vi "sc5511a_soft_front_panel.vi"() -> ()   [LabVIEW 2010]
panel:
  out "message":string="List/Sweep Mode Disabled"
  out "On":bool
  in  "stop":bool
  in  "Tab Control":T1(tab)
  in  "Spur Suppression":u8(ring) items=["Enabled", "Disabled"]
  in  "AutoLevel":u8(ring) items=["Enable", "Disable"]
  in  "Loop Gain":u8(ring) items=["Normal", "Low"]
  in  "Ref. Out Freq":u8(ring) items=["10 MHz", "100 MHz"]
  in  "Ref. Clock Source":u8(ring) items=["Internal 10 MHz", "Lock to External"]
  in  "RF1 Standby":bool
  in  "Lock Mode":u8(ring) items=["Harmonic Lock", "Frac-N Lock"]
  in  "ALC MODE":u8(ring) items=["Closed", "Opened"]
  in  "Power":sgl=30.0 min=-40 max=30 format="%.2f"
  in  "Interval (s)":u16=5
  in  "GetStatus":bool
  in  "Trigger":bool
  out "Device Status":T2={"Synth Mode"=1, "RF Out"=0, "Auto Level"=0, "ALC Mode"=1, "Standby"=1, "Rf RF Mode"=0, "List Mode State"=0, "RF2 Standby"=0, "Ref Lock Enable"=1, "Ext Ref Detected"=1, "Ref out mode"=1, "Main PLL"=1, "Crs PLL"=1, "Fine PLL"=1, "device accessed"=0, "Over Temp"=0, "MainLED"=FALSE, "CrsLED"=FALSE, "FineLED"=FALSE} {"Over Temp" items=["Normal", "Over Temp"]; "Ref out mode" items=["10 MHz", "100 MHz"]; "device accessed" items=["NO", "YES"]; "RF2 Standby" items=["Disabled", "Enabled"]; "Standby" items=["Disable", "Enabled"]; "Auto Level" items=["Enable", "Disable"]; "Ext Ref Detected" items=["Not Detected", "Detected"]; "Ref Lock Enable" items=["Disabled", "Enabled"]; "RF Out" items=["Disabled", "Enabled"]; "ALC Mode" items=["Closed", "Opened"]; "Rf RF Mode" items=["Single Tone", "List/Sweep"]; "Synth Mode" items=["Harmonic", "FracN"]; "List Mode State" items=["Not Triggered", "Triggered"]; "Main PLL" items=["NOT Locked", "Locked"]; "Crs PLL" items=["NOT Locked", "Locked"]; "Fine PLL" items=["NOT Locked", "Locked"]}
  in  "RF Frequency":dbl=2005000000.0 min=80000000.0 max=21000000000.0 step=1.0 format="%.9p"
  in  "RF Mode":u8(ring) items=["Single Tone", "List/Sweep"]
  in  "RF Enable":bool
  in  "RF2 Freq":sgl=6000.0 min=25 max=6000 step=25
  in  "RF2 Standby":bool
  in  "Set As Default":bool
  in  "Dwell Period (ms)":dbl=10.0 min=0.0 step=0.5 format="%.1f"
  in  "Sweep/List Cycles":u32
  in  "Sweep Freq Parameter":T3={"Start Frequency"=10040000000, "Stop Frequency"=10050000000, "Step Frequency"=100000} {"Step Frequency" max=6500000000 format="%.9p"; "Stop Frequency" max=21000000000 format="%.9p"; "Start Frequency" format="%.9p"}
  in  "List Mode Config":T4={"Sweep / List"=1, "Direction"=0, "Shape"=1, "Trigger Source"=1, "HW Trigger Mode"=0, "Return to Start"=0, "Trigger Out State"=1, "Trigger Out Behavior"=0} {"Trigger Out Behavior" items=["Trigger On Step", "Trigger On Cycle"]; "Trigger Out State" items=["Trigger Out Disable", "Trigger Out Enable"]; "Return to Start" items=["Stop at End", "Return to Start"]; "HW Trigger Mode" items=["Start/Stop", "Step"]; "Trigger Source" items=["Software", "Hardware"]; "Shape" items=["Sawtooth", "Triangle"]; "Direction" items=["Low to High", "High to Low"]; "Sweep / List" items=["List", "Sweep (start/stop/step)"]}
  in  "Load Config":bool
  in  "Save Buffer to EEPROM":bool
  in  "Read EEPROM to Buffer":bool
  in  "Download to Buffer":bool
  in  "Read From File":bool
  in  "Frequency List (2048 max)":u64[](array[numeric]) format="%.9p"
  out "message 2":string
  out "List Points":u32
  in  "SelfCal":bool
  out "Temperature":sgl=40.0 min=-30 max=120 format="%.1f"
  out "Device Info":T5={"Product SN"=268435879, "Hardware Rev"=2.0, "Firmware Rev"=2.0, "Manuf Date"={"Year"=14, "Month"=9, "Day"=10, "Hour"=10}} {"Firmware Rev" format="%.2g"; "Hardware Rev" format="%.2g"; "Product SN" format="%.0x"}
  out "error out":errorcluster
  # "MHz"
  # "Program will stop and the device will \nreinitialize after self calibration"
  # "DegC"
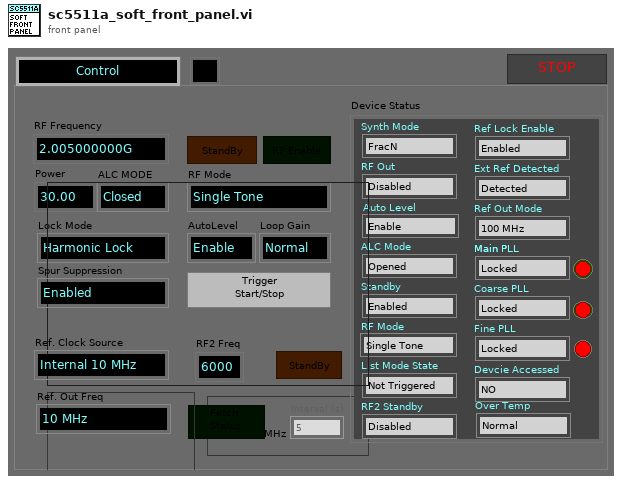
[diagram p1: front panel]
types:
  T1 = enum32{"Control", "Config Sweep/List", "List Entry", "Device Info"}
  T2 = cluster{"Synth Mode":u16, "RF Out":u16, "Auto Level":u16, "ALC Mode":u16, "Standby":u16, "Rf RF Mode":u16, "List Mode State":u16, "RF2 Standby":u16, "Ref Lock Enable":u16, "Ext Ref Detected":u16, "Ref out mode":u16, "Main PLL":u8, "Crs PLL":u8, "Fine PLL":u8, "device accessed":u16, "Over Temp":u16, "MainLED":bool, "CrsLED":bool, "FineLED":bool}
  T3 = cluster{"Start Frequency":u64, "Stop Frequency":u64, "Step Frequency":u64}
  T4 = cluster{"Sweep / List":u8, "Direction":u8, "Shape":u8, "Trigger Source":u8, "HW Trigger Mode":u8, "Return to Start":u8, "Trigger Out State":u8, "Trigger Out Behavior":u8}
  T5 = cluster{"Product SN":u32, "Hardware Rev":sgl, "Firmware Rev":sgl, "Manuf Date":cluster{"Year":u8, "Month":u8, "Day":u8, "Hour":u8}}
  T6 = cluster{"Product SN":u32, "Hardware Rev":sgl, "Firmware Rev":sgl, "Manuf Date":cluster{"Year":u32, "Month":u32, "Day":u32, "hour":u32}}
  T7 = enum32{"Control", "Config Sweep/List", "List Entry"}
  T8 = enum8{"Enabled", "Disabled", "Disabled and Grayed Out"}
  T9 = cluster{"Synth Mode":u16, "RF Out":u16, "Auto Power":u16, "ALC Mode":u16, "Standby":u16, "Rf RF Mode":u16, "List Mode State":u16, "RF2 Standby":u16, "Ref Lock Enable":u16, "Ext Ref Detected":u16, "Ref out mode":u16, "Main PLL":u8, "Crs PLL":u8, "Fine PLL":u8, "device accessed":u16, "Over Temp":u16, "MainLED":bool, "CrsLED":bool, "FineLED":bool}
  T10 = cluster{"Product SN":u32, "Hardware Rev":sgl, "Firmware Rev":sgl, "Manufacture Date":cluster{"Year":u8, "Month":u8, "Day":u8, "hour":u8}}
  T11 = cluster{"List Mode Config":cluster{"List/SSS":u8, "Direction":u8, "Shape":u8, "Trigger Source":u8, "HW Trigger Mode":u8, "Return to Start":u8, "Trigger Out State":u8, "Trigger Out Behavior":u8}, "Operate Status":cluster{"Lock Mode":u8, "Loop Gain":u8, "Device Accessed":u8, "RF2 Standby":u8, "RF1 Standby":u8, "AutoPwrLevel":u8, "AlcMode":u8, "RFOutState":u8, "Ref Lock Enable":u8, "ExtRefDetected":u8, "RefOutSelect":u8, "ListRuning":u8, "RF Mode":u8, "OverTempStatus":u8, "Harmonic SS":u8}, "PLL Status":cluster{"Sum PLL":u8, "Crs PLL":u8, "Fine PLL":u8, "Crs Ref PLL":u8, "Crs assist PLL":u8, "Ref Clk PLL":u8, "Clk 10 PLL":u8, "Lo2 PLL":u8}}
  T12 = cluster{"RF1 Freq":u64, "Sweep Start Freq":u64, "Sweep Stop Freq":u64, "Sweep Step Freq":u64, "Sweep dwell time (.5ms)":u32, "Sweep Cycles":u32, "List Buffer Points":u32, "RF1 Level (dBm)":sgl, "RF2 freq":u16}
  T13 = cluster{"List/SSS":u8, "Direction":u8, "Shape":u8, "Trigger Source":u8, "HW Trigger Mode":u8, "Return to Start":u8, "Trigger Out State":u8, "Trigger Out Behavior":u8}
  T14 = cluster{"Sweep Start Freq":u64, "Sweep Stop Freq":u64, "Sweep Step Freq":u64}
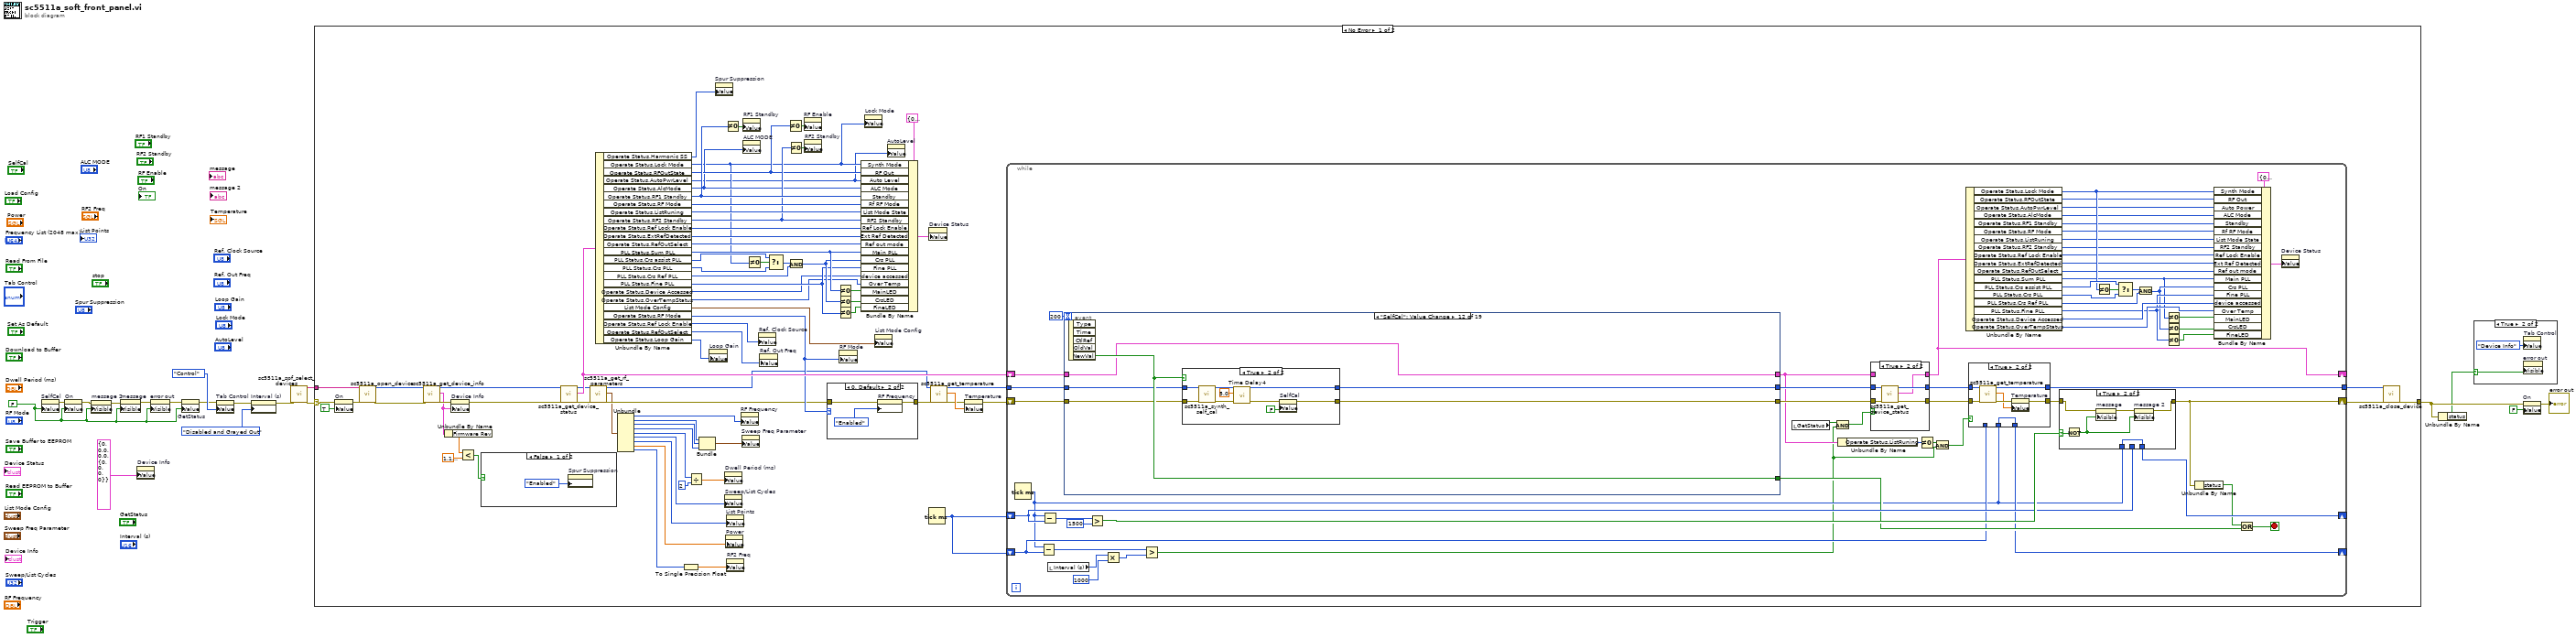
[diagram p0: block diagram]
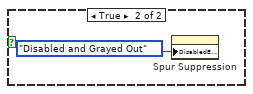
[diagram p3: hidden frame]
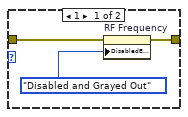
[diagram p4: hidden frame]
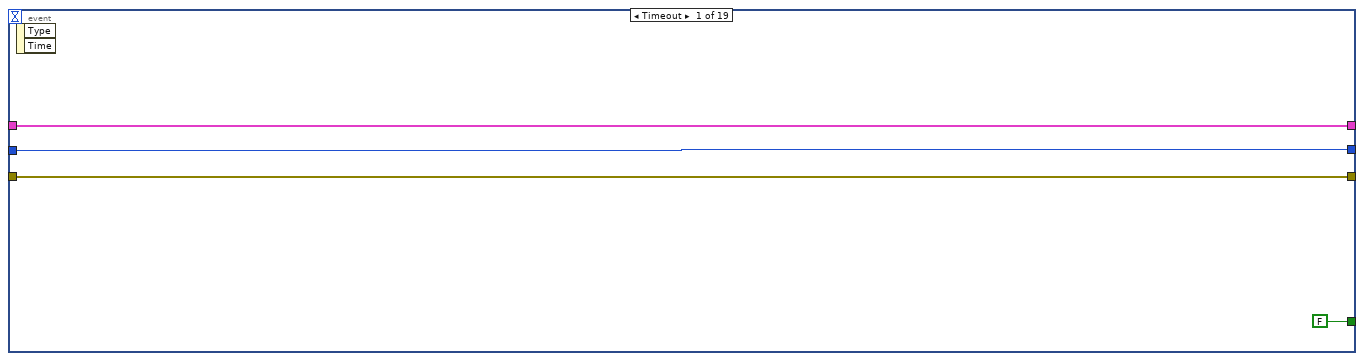
[diagram p8: hidden frame]
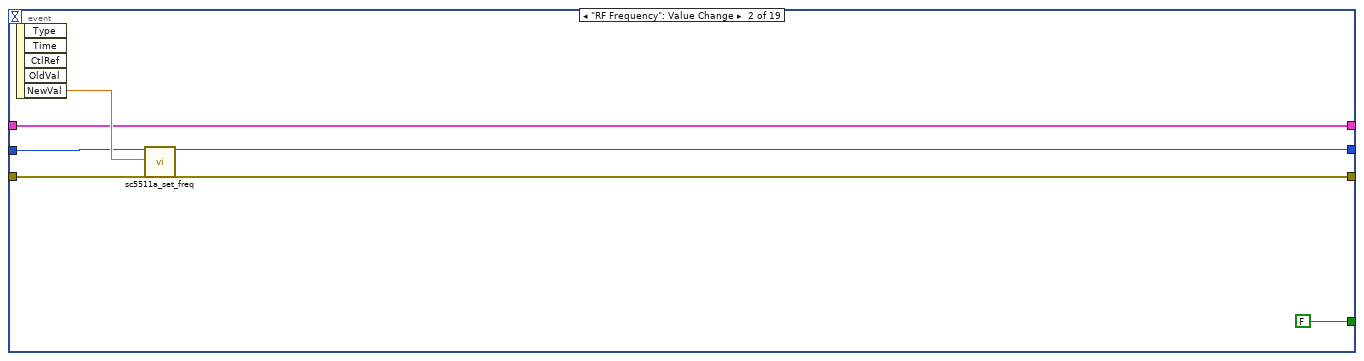
[diagram p9: hidden frame]
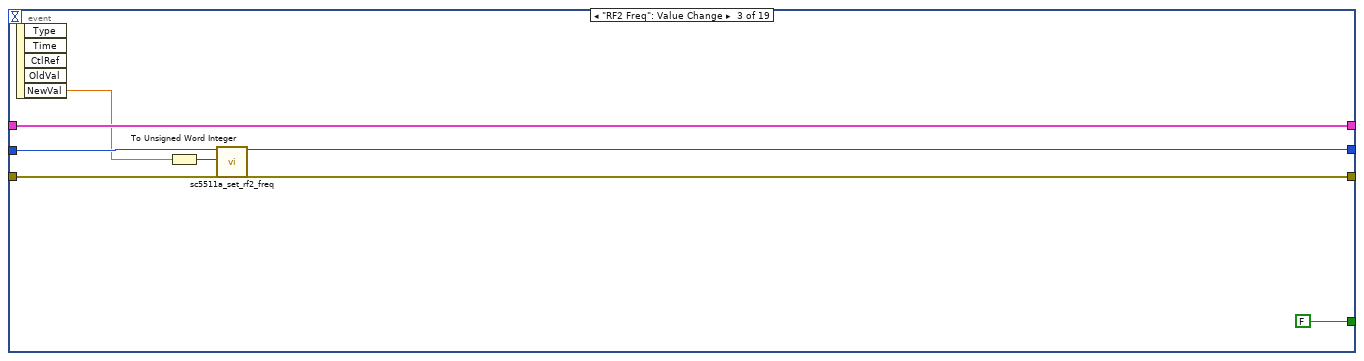
[diagram p10: hidden frame]
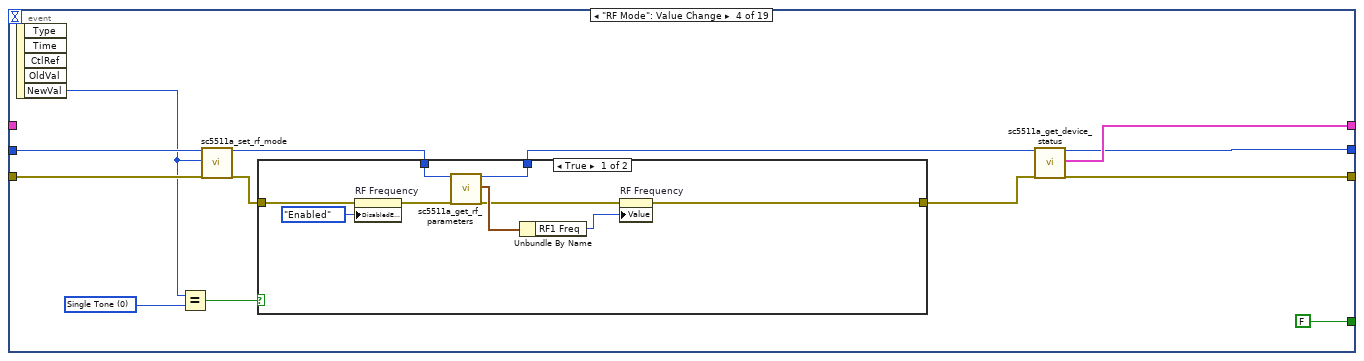
[diagram p11: hidden frame]
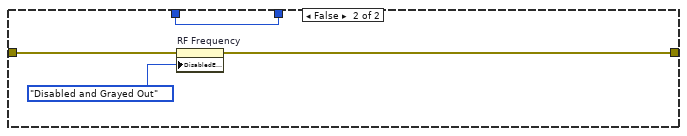
[diagram p12: hidden frame]
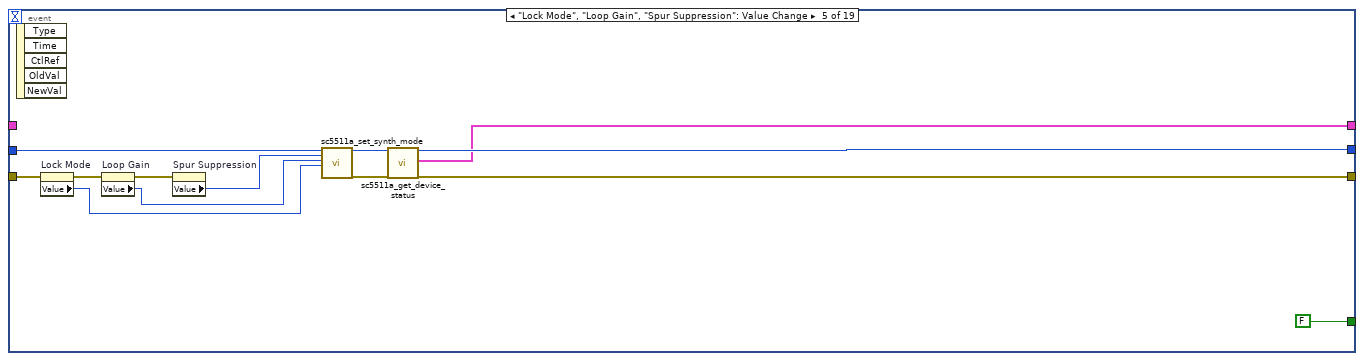
[diagram p13: hidden frame]
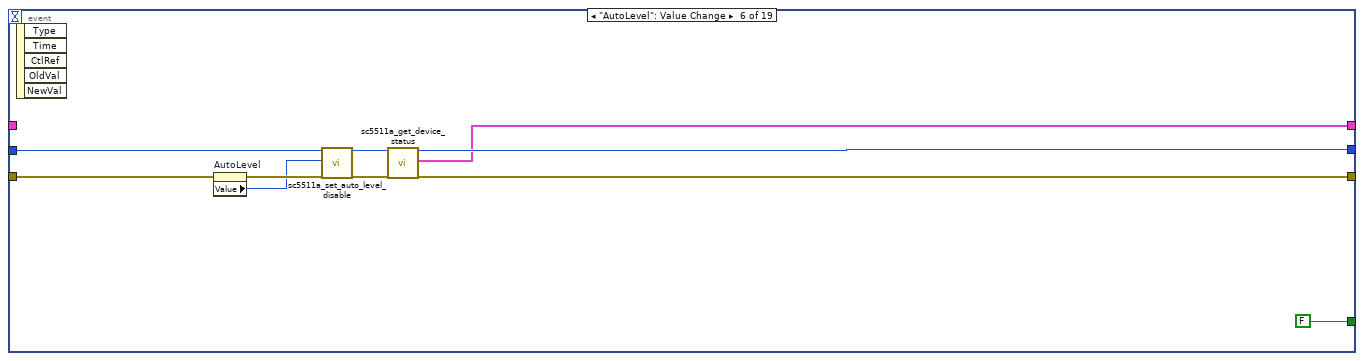
[diagram p14: hidden frame]
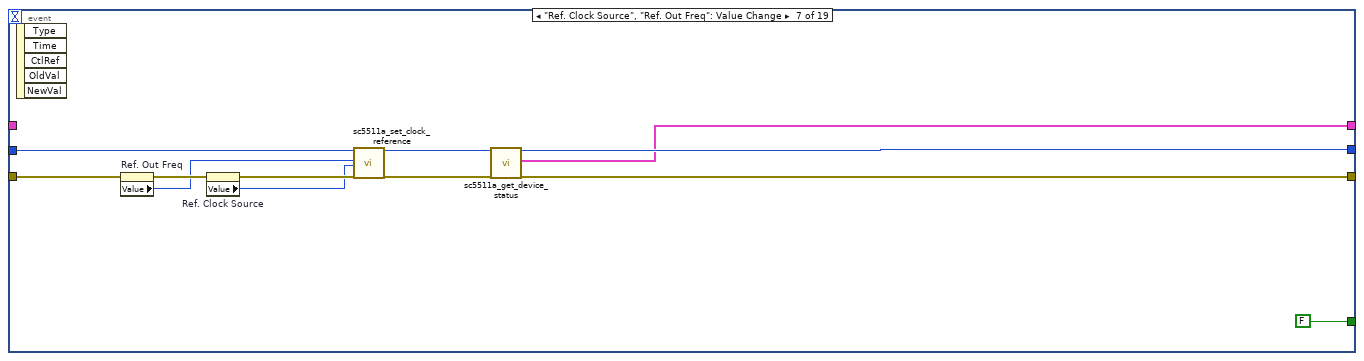
[diagram p15: hidden frame]
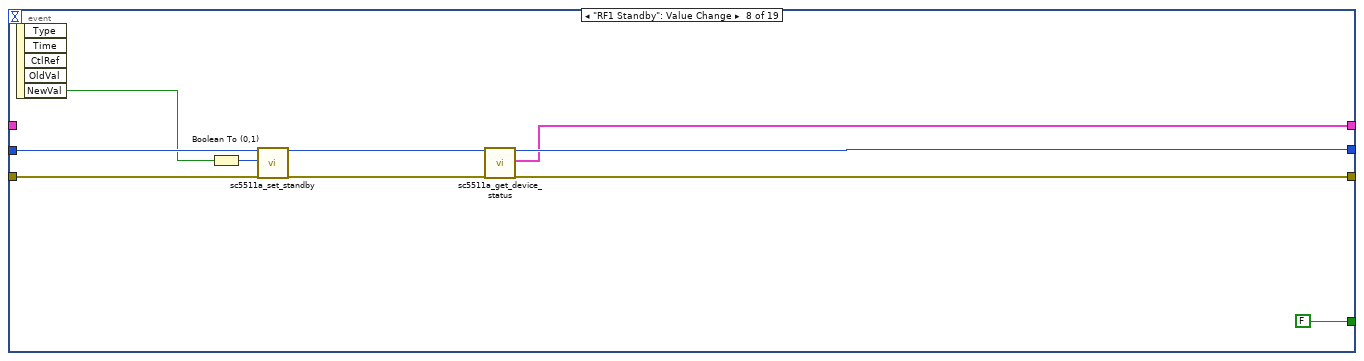
[diagram p16: hidden frame]
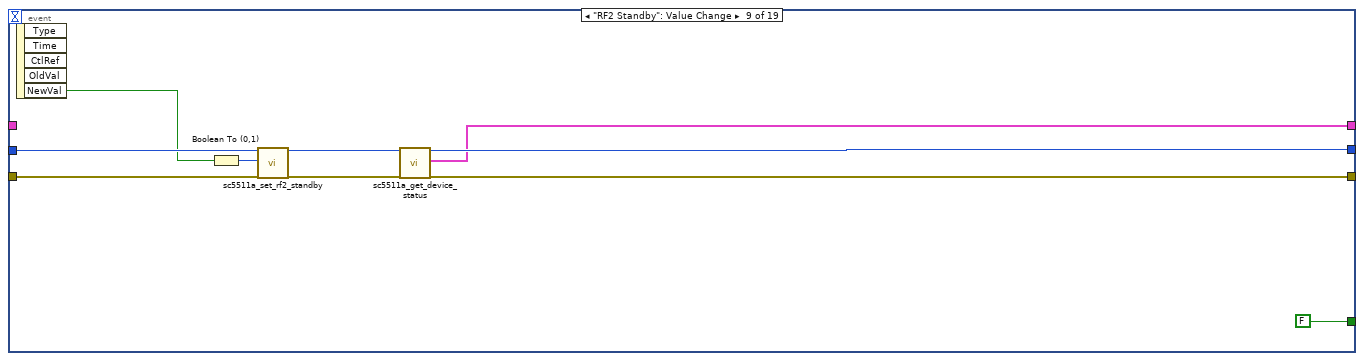
[diagram p17: hidden frame]
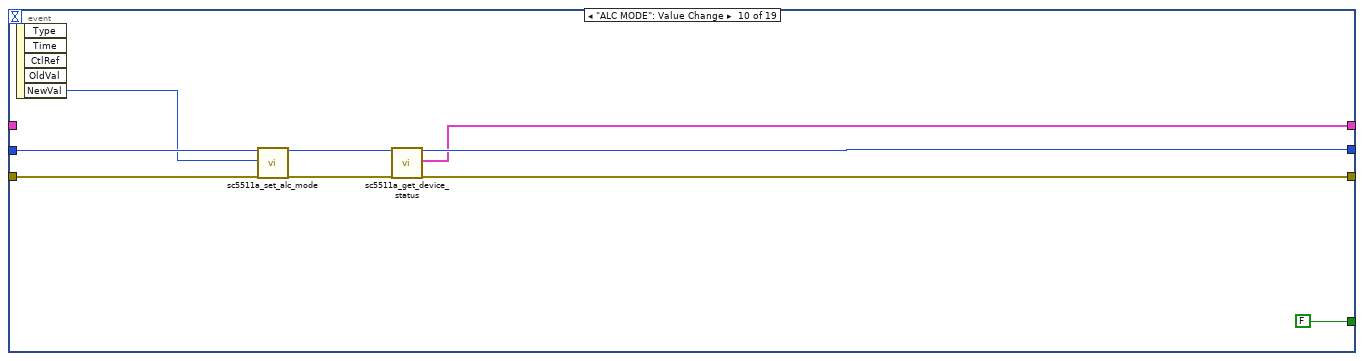
[diagram p18: hidden frame]
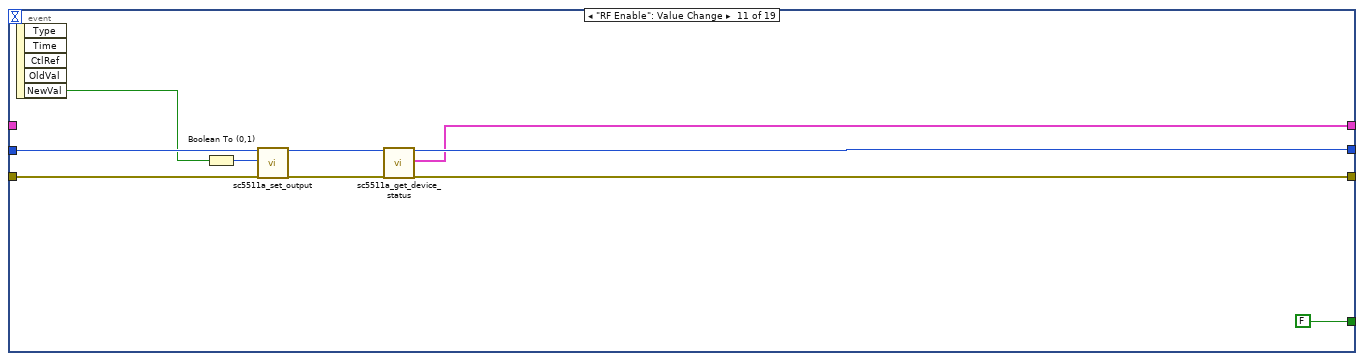
[diagram p19: hidden frame]
diagram:
  w1 = FALSE ("Visible")
  n1 = property on="SelfCal" class="Bool (strict)"("Value"=w1) -> (error out=w2:errorcluster)  [unwired: 2 in, 1 out]
  n2 = property on="On" class="Bool (strict)"(error in=w2, "Value"=w1) -> (error out=w4:errorcluster)  [unwired: 1 in, 1 out]
  n3 = property on="message 2" class="Str"(error in=w4, "Visible"=w1) -> (error out=w18:errorcluster)  [unwired: 1 in, 1 out]
  n4 = property on="message" class="Str"(error in=w18, "Visible"=w1) -> (error out=w17:errorcluster)  [unwired: 1 in, 1 out]
  n5 = property on="Device Info" class="Clust (strict)"("Value"=T6 {"Product SN"=0, "Hardware Rev"=0.0, "Firmware Rev"=0.0, "Manuf Date"={"Year"=0, "Month"=0, "Day"=0, "hour"=0}} ("Device Info")) -> ()  [unwired: 2 in, 2 out]
  n6 = property on="error out" class="Clust (strict)"(error in=w17, "Visible"=w1) -> (error out=w15:errorcluster)  [unwired: 1 in, 1 out]
  n7 = property on="GetStatus" class="Bool (strict)"(error in=w15, "Value"=w1) -> (error out=w10:errorcluster)  [unwired: 1 in, 1 out]
  n8 = property on="Tab Control" class="TabCtl (strict)"(error in=w10, "Value"=T7."Control" ("Tab Control")) -> (error out=w11:errorcluster)  [unwired: 1 in, 1 out]
  n9 = property on="Interval (s)" class="DigNum (strict)"(error in=w11, "DisabledEnum"=T8."Disabled and Grayed Out" ("Disabled")) -> (error out=w14:errorcluster)  [unwired: 1 in, 1 out]
  n10 = call "sc5511a_spf_select_devices.vi"("error in (no error)"=w14) -> ("Selected Resource"=w8:string, "error out"=w16:errorcluster)  [unwired: 17 in]
  n11 = case shown="No Error" w16 {
    selector: w16 -> [w78 w552]
    tunnel: [w92 w552] -> w7
    tunnel: w8 -> [w77 _]
    frame No Error {
      n12 = property on="On" class="Bool (strict)"(error in=w78, "Value"=TRUE ("Visible")) -> (error out=w79:errorcluster)  [unwired: 1 in, 1 out]
      n13 = call "sc5511a_open_device.vi"("Device SN String"=w77, "error in (no error)"=w79) -> ("deviceHandle"=w81:u32, "error out"=w82:errorcluster)  [unwired: 16 in]
      n14 = call "sc5511a_get_device_info.vi"("deviceHandle"=w81, "error in"=w82) -> ("deviceHandle"=w89:u32, "Device Info"=w22:T10, "error out"=w88:errorcluster)  [unwired: 15 in]
      n15 = Unbundle By Name(w22) -> ("Firmware Rev"=w21:sgl)
      n16 = property on="Device Info" class="Clust (strict)"(error in=w88, "Value"=w22) -> (error out=w87:errorcluster)  [unwired: 1 in, 1 out]
      n17 = Less?(x=w21, y=sgl 1.1) -> (x < y?=w19:bool)
      n18 = case shown="False" w19 {
        frame False {
          n19 = property on="Spur Suppression" class="Ring (strict)"("DisabledEnum"=T8."Enabled" ("Disabled")) -> ()  [unwired: 2 in, 2 out]
        }
        frame True {
          n20 = property on="Spur Suppression" class="Ring (strict)"("DisabledEnum"=T8."Disabled and Grayed Out" ("Disabled")) -> ()  [unwired: 2 in, 2 out]
        }
      }
      n21 = call "sc5511a_get_device_status.vi"("deviceHandle"=w89, "error in"=w87) -> ("deviceHandle"=w73:u32, "Device Status"=w90:T11, "error out"=w75:errorcluster)  [unwired: 15 in]
      n22 = call "sc5511a_get_rf_parameters.vi"("deviceHandle"=w73, "error in"=w75) -> ("deviceHandle"=w34:u32, "RF Params"=w72:T12, "error out"=w74:errorcluster)  [unwired: 15 in]
      n23 = Unbundle By Name(w90) -> ("Operate Status.Harmonic SS"=w23:u8, "Operate Status.Lock Mode"=w27:u8, "Operate Status.RFOutState"=w36:u8, "Operate Status.AutoPwrLevel"=w24:u8, "Operate Status.AlcMode"=w35:u8, "Operate Status.RF1 Standby"=w41:u8, "Operate Status.RF Mode"=w58:u8, "Operate Status.ListRuning"=w57:u8, "Operate Status.RF2 Standby"=w37:u8, "Operate Status.Ref Lock Enable"=w56:u8, "Operate Status.ExtRefDetected"=w55:u8, "Operate Status.RefOutSelect"=w54:u8, "PLL Status.Sum PLL"=w53:u8, "PLL Status.Crs assist PLL"=w49:u8, "PLL Status.Crs PLL"=w48:u8, "PLL Status.Crs Ref PLL"=w50:u8, "PLL Status.Fine PLL"=w46:u8, "Operate Status.Device Accessed"=w45:u8, "Operate Status.OverTempStatus"=w44:u8, "List Mode Config"=w91:T13, "Operate Status.RF Mode"=w80:u8, "Operate Status.Ref Lock Enable"=w43:u8, "Operate Status.RefOutSelect"=w42:u8, "Operate Status.Loop Gain"=w28:u8)
      n24 = Unbundle(w72) -> ("RF1 Freq"=w71:u64, "Sweep Start Freq"=w69:u64, "Sweep Stop Freq"=w68:u64, "Sweep Step Freq"=w67:u64, "Sweep dwell time (.5ms)"=w64:u32, "Sweep Cycles"=w66:u32, "List Buffer Points"=w62:u32, "RF1 Level (dBm)"=w61:sgl, "RF2 freq"=w59:u16)
      n25 = To Single Precision Float(number=w59) -> (single precision float=w60:sgl)
      n26 = Divide(x=w64, y=u32 2) -> (x/y=w65:dbl)
      n27 = Bundle("Sweep Start Freq"=w69, "Sweep Stop Freq"=w68, "Sweep Step Freq"=w67) -> (w70:T14)  [unwired: 1 in]
      n28 = property on="Loop Gain" class="Ring (strict)"("Value"=w28) -> ()  [unwired: 2 in, 2 out]
      n29 = property on="Spur Suppression" class="Ring (strict)"("Value"=w23) -> ()  [unwired: 2 in, 2 out]
      n30 = Not Equal To 0?(x=w41) -> (x != 0?=w40:bool)
      n31 = property on="Dwell Period (ms)" class="DigNum (strict)"("Value"=w65) -> ()  [unwired: 2 in, 2 out]
      n32 = property on="Sweep/List Cycles" class="DigNum (strict)"("Value"=w66) -> ()  [unwired: 2 in, 2 out]
      n33 = property on="Power" class="DigNum (strict)"("Value"=w61) -> ()  [unwired: 2 in, 2 out]
      n34 = property on="List Points" class="DigNum (strict)"("Value"=w62) -> ()  [unwired: 2 in, 2 out]
      n35 = property on="RF2 Freq" class="DigNum (strict)"("Value"=w60) -> ()  [unwired: 2 in, 2 out]
      n36 = property on="RF Frequency" class="DigNum (strict)"("Value"=w71) -> ()  [unwired: 2 in, 2 out]
      n37 = property on="Sweep Freq Parameter" class="Clust (strict)"("Value"=w70) -> ()  [unwired: 2 in, 2 out]
      n38 = property on="RF1 Standby" class="Bool (strict)"("Value"=w40) -> ()  [unwired: 2 in, 2 out]
      n39 = property on="ALC MODE" class="Ring (strict)"("Value"=w35) -> ()  [unwired: 2 in, 2 out]
      n40 = Not Equal To 0?(x=w27) -> (x != 0?=w52:bool)
      n41 = property on="Ref. Clock Source" class="Ring (strict)"("Value"=w43) -> ()  [unwired: 2 in, 2 out]
      n42 = property on="Ref. Out Freq" class="Ring (strict)"("Value"=w42) -> ()  [unwired: 2 in, 2 out]
      n43 = Select(t=w49, s=w52, f=w48) -> (s? t:f=w51:u8)
      n44 = Not Equal To 0?(x=w36) -> (x != 0?=w39:bool)
      n45 = Not Equal To 0?(x=w37) -> (x != 0?=w38:bool)
      n46 = And(x=w51, y=w50) -> (x .and. y?=w47:u8)
      n47 = property on="RF Enable" class="Bool (strict)"("Value"=w39) -> ()  [unwired: 2 in, 2 out]
      n48 = property on="RF2 Standby" class="Bool (strict)"("Value"=w38) -> ()  [unwired: 2 in, 2 out]
      n49 = case shown="0, Default" w80 {
        tunnel: w74 -> [w98 w101]
        tunnel: [w97 w100] -> w32
        frame 1 {
          n50 = property on="RF Frequency" class="DigNum (strict)"(error in=w98, "DisabledEnum"=T8."Disabled and Grayed Out" ("Disabled")) -> (error out=w97:errorcluster)  [unwired: 1 in, 1 out]
        }
        frame 0, Default {
          n51 = property on="RF Frequency" class="DigNum (strict)"(error in=w101, "DisabledEnum"=T8."Enabled" ("Disabled")) -> (error out=w100:errorcluster)  [unwired: 1 in, 1 out]
        }
      }
      n52 = Not Equal To 0?(x=w53) -> (x != 0?=w85:bool)
      n53 = Not Equal To 0?(x=w47) -> (x != 0?=w84:bool)
      n54 = Not Equal To 0?(x=w46) -> (x != 0?=w83:bool)
      n55 = property on="RF Mode" class="Ring (strict)"("Value"=w80) -> ()  [unwired: 2 in, 2 out]
      n56 = Bundle By Name(cluster=T2 {"Synth Mode"=0, "RF Out"=1, "Auto Level"=1, "ALC Mode"=0, "Standby"=0, "Rf RF Mode"=0, "List Mode State"=0, "RF2 Standby"=1, "Ref Lock Enable"=0, "Ext Ref Detected"=0, "Ref out mode"=0, "Main PLL"=1, "Crs PLL"=1, "Fine PLL"=1, "device accessed"=1, "Over Temp"=0, "MainLED"=TRUE, "CrsLED"=TRUE, "FineLED"=TRUE} ("Device Status"), "Synth Mode"=w27, "RF Out"=w36, "Auto Level"=w24, "ALC Mode"=w35, "Standby"=w41, "Rf RF Mode"=w58, "List Mode State"=w57, "RF2 Standby"=w37, "Ref Lock Enable"=w56, "Ext Ref Detected"=w55, "Ref out mode"=w54, "Main PLL"=w53, "Crs PLL"=w47, "Fine PLL"=w46, "device accessed"=w45, "Over Temp"=w44, "MainLED"=w85, "CrsLED"=w84, "FineLED"=w83) -> (w26:T2)
      n57 = property on="Lock Mode" class="Ring (strict)"("Value"=w27) -> ()  [unwired: 2 in, 2 out]
      n58 = property on="List Mode Config" class="Clust (strict)"("Value"=w91) -> ()  [unwired: 2 in, 2 out]
      n59 = property on="AutoLevel" class="Ring (strict)"("Value"=w24) -> ()  [unwired: 2 in, 2 out]
      n60 = Tick Count (ms)() -> (millisecond timer value=w86:u32)
      n61 = property on="Device Status" class="Clust (strict)"("Value"=w26) -> ()  [unwired: 2 in, 2 out]
      n62 = call "sc5511a_get_temperature.vi"("deviceHandle"=w34, "error in"=w32) -> ("deviceHandle"=w33:u32, "temperature"=w31:sgl, "error out"=w29:errorcluster)  [unwired: 15 in]
      n63 = property on="Temperature" class="DigNum (strict)"(error in=w29, "Value"=w31) -> (error out=w30:errorcluster)  [unwired: 1 in, 1 out]
      n64 = while {
        shift-right: [w144] -> w94
        shift-left: w30 -> [w162]
        tunnel: w33 -> [w161]
        tunnel: [w111] -> w93
        shift-right: [w119] -> _
        shift-left: w90 -> [w158]
        shift-right: [w148] -> _
        shift-left: w86 -> [w147]
        shift-right: [w114] -> _
        shift-left: w86 -> [w115]
        stop <- w143 stop-if-true
        n65 = Tick Count (ms)() -> (millisecond timer value=w113:u32)
        n66 = Subtract(x=w113, y=w115) -> (x-y=w152:u32)
        n67 = Subtract(x=w113, y=w147) -> (x-y=w157:u32)
        n68 = local read "Interval (s)"() -> (w153:u16)
        n69 = event shown="[11] \"SelfCal\": Value Change" {
          selector: _ -> [_ _ _ _ _ _ _ _ _ _ _ _ _ _ _ _ _ _ _]
          dyn-events: _ -> [_ _ _ _ _ _ _ _ _ _ _ _ _ _ _ _ _ _ _]
          timeout: 200 -> [_ _ _ _ _ _ _ _ _ _ _ _ _ _ _ _ _ _ _]
          tunnel: w161 -> [w191 w198 w207 w218 w245 w255 w267 w276 w286 w295 w305 w312 w327 w332 w353 w364 w436 w451 w498]
          tunnel: w162 -> [w192 w197 w206 w219 w239 w247 w266 w277 w287 w296 w306 w311 w328 w337 w350 w365 w435 w452 w499]
          tunnel: [w191 w195 w204 w210 w242 w252 w258 w271 w282 w291 w300 w308 w326 w333 w353 w357 w412 w450 w493] -> w160
          tunnel: [w192 w196 w205 w211 w244 w254 w261 w272 w283 w293 w302 w309 w325 w334 w351 w359 w410 w449 w494] -> w159
          tunnel: w158 -> [w190 w194 w203 _ _ _ _ _ _ _ _ w310 w330 _ w354 w360 w408 w444 w491]
          tunnel: [w190 w194 w203 w213 w240 w250 w257 w269 w279 w289 w298 w310 w330 w331 w354 w355 w408 w444 w491] -> w108
          tunnel: [FALSE ("NewVal") FALSE FALSE FALSE FALSE FALSE FALSE FALSE FALSE FALSE FALSE w313 FALSE FALSE TRUE ("NewVal") FALSE ("NewVal") FALSE ("NewVal") FALSE ("NewVal") FALSE ("NewVal")] -> w146
          event Timeout {
            n70 = event-data() -> ()  [unwired: 1 in, 2 out]
          }
          event "RF Frequency": Value Change {
            n71 = event-data() -> ("NewVal"=w199:dbl)  [unwired: 1 in, 4 out]
            n72 = call "sc5511a_set_freq.vi"("deviceHandle"=w198, "RF1 frequency"=w199, "error in"=w197) -> ("deviceHandle"=w195:u32, "error out"=w196:errorcluster)  [unwired: 15 in]
          }
          event "RF2 Freq": Value Change {
            n73 = event-data() -> ("NewVal"=w200:sgl)  [unwired: 1 in, 4 out]
            n74 = To Unsigned Word Integer(number=w200) -> (unsigned 16bit integer=w201:u16)
            n75 = call "sc5511a_set_rf2_freq.vi"("deviceHandle"=w207, "RF1 frequency (MHz)"=w201, "error in"=w206) -> ("deviceHandle"=w204:u32, "error out"=w205:errorcluster)  [unwired: 15 in]
          }
          event "RF Mode": Value Change {
            w216 = u8 0 items=["Single Tone", "List/Sweep"] ("RF Mode")
            n76 = event-data() -> ("NewVal"=w215:u8)  [unwired: 1 in, 4 out]
            n77 = Equal?(x=w215, y=w216) -> (x = y?=w214:bool)
            n78 = call "sc5511a_set_rf_mode.vi"("deviceHandle"=w218, "RF Mode"=w215, "error in"=w219) -> ("deviceHandle"=w209:u32, "error out"=w217:errorcluster)  [unwired: 15 in]
            n79 = case shown="True" w214 {
              tunnel: w217 -> [w229 w233]
              tunnel: [w221 w232] -> w212
              tunnel: w209 -> [w226 w230]
              tunnel: [w225 w230] -> w208
              frame True {
                n80 = property on="RF Frequency" class="DigNum (strict)"(error in=w229, "DisabledEnum"=T8."Enabled" ("Disabled")) -> (error out=w227:errorcluster)  [unwired: 1 in, 1 out]
                n81 = call "sc5511a_get_rf_parameters.vi"("deviceHandle"=w226, "error in"=w227) -> ("deviceHandle"=w225:u32, "RF Params"=w224:T12, "error out"=w222:errorcluster)  [unwired: 15 in]
                n82 = Unbundle By Name(w224) -> ("RF1 Freq"=w223:u64)
                n83 = property on="RF Frequency" class="DigNum (strict)"(error in=w222, "Value"=w223) -> (error out=w221:errorcluster)  [unwired: 1 in, 1 out]
              }
              frame False {
                n84 = property on="RF Frequency" class="DigNum (strict)"(error in=w233, "DisabledEnum"=T8."Disabled and Grayed Out" ("Disabled")) -> (error out=w232:errorcluster)  [unwired: 1 in, 1 out]
              }
            }
            n85 = call "sc5511a_get_device_status.vi"("deviceHandle"=w208, "error in"=w212) -> ("deviceHandle"=w210:u32, "Device Status"=w213:T11, "error out"=w211:errorcluster)  [unwired: 15 in]
          }
          event "Lock Mode", "Loop Gain", "Spur Suppression": Value Change {
            n86 = event-data() -> ()  [unwired: 1 in, 5 out]
            n87 = property on="Lock Mode" class="Ring (strict)"(error in=w239) -> (error out=w238:errorcluster, "Value"=w236:u8)  [unwired: 1 in, 1 out]
            n88 = property on="Loop Gain" class="Ring (strict)"(error in=w238) -> (error out=w235:errorcluster, "Value"=w237:u8)  [unwired: 1 in, 1 out]
            n89 = property on="Spur Suppression" class="Ring (strict)"(error in=w235) -> ("Value"=w234:u8)  [unwired: 1 in, 2 out]
            n90 = call "sc5511a_set_synth_mode.vi"("deviceHandle"=w245, "Harmonic Spur Suppression"=w234, "loop gain"=w237, "lock mode"=w236) -> ("deviceHandle"=w241:u32, "error out"=w243:errorcluster)  [unwired: 14 in]
            n91 = call "sc5511a_get_device_status.vi"("deviceHandle"=w241, "error in"=w243) -> ("deviceHandle"=w242:u32, "Device Status"=w240:T11, "error out"=w244:errorcluster)  [unwired: 15 in]
          }
          event "AutoLevel": Value Change {
            n92 = event-data() -> ()  [unwired: 1 in, 5 out]
            n93 = property on="AutoLevel" class="Ring (strict)"(error in=w247) -> (error out=w249:errorcluster, "Value"=w248:u8)  [unwired: 1 in, 1 out]
            n94 = call "sc5511a_set_auto_level_disable.vi"("deviceHandle"=w255, "auto leveling"=w248, "error in"=w249) -> ("deviceHandle"=w251:u32, "error out"=w253:errorcluster)  [unwired: 15 in]
            n95 = call "sc5511a_get_device_status.vi"("deviceHandle"=w251, "error in"=w253) -> ("deviceHandle"=w252:u32, "Device Status"=w250:T11, "error out"=w254:errorcluster)  [unwired: 15 in]
          }
          event "Ref. Clock Source", "Ref. Out Freq": Value Change {
            n96 = event-data() -> ()  [unwired: 1 in, 5 out]
            n97 = property on="Ref. Out Freq" class="Ring (strict)"(error in=w266) -> (error out=w265:errorcluster, "Value"=w262:u8)  [unwired: 1 in, 1 out]
            n98 = property on="Ref. Clock Source" class="Ring (strict)"(error in=w265) -> (error out=w264:errorcluster, "Value"=w263:u8)  [unwired: 1 in, 1 out]
            n99 = call "sc5511a_set_clock_reference.vi"("deviceHandle"=w267, "Ref Output"=w262, "Lock external"=w263, "error in"=w264) -> ("deviceHandle"=w259:u32, "error out"=w260:errorcluster)  [unwired: 14 in]
            n100 = call "sc5511a_get_device_status.vi"("deviceHandle"=w259, "error in"=w260) -> ("deviceHandle"=w258:u32, "Device Status"=w257:T11, "error out"=w261:errorcluster)  [unwired: 15 in]
          }
          event "RF1 Standby": Value Change {
            n101 = event-data() -> ("NewVal"=w275:bool)  [unwired: 1 in, 4 out]
            n102 = Boolean To (0,1)(Boolean=w275) -> (0, 1=w274:i16)
            n103 = call "sc5511a_set_standby.vi"("deviceHandle"=w276, "Standby"=w274, "error in"=w277) -> ("deviceHandle"=w270:u32, "error out"=w273:errorcluster)  [unwired: 15 in]
            n104 = call "sc5511a_get_device_status.vi"("deviceHandle"=w270, "error in"=w273) -> ("deviceHandle"=w271:u32, "Device Status"=w269:T11, "error out"=w272:errorcluster)  [unwired: 15 in]
          }
          event "RF2 Standby": Value Change {
            n105 = event-data() -> ("NewVal"=w285:bool)  [unwired: 1 in, 4 out]
            n106 = Boolean To (0,1)(Boolean=w285) -> (0, 1=w284:i16)
            n107 = call "sc5511a_set_rf2_standby.vi"("deviceHandle"=w286, "Standby"=w284, "error in"=w287) -> ("deviceHandle"=w281:u32, "error out"=w280:errorcluster)  [unwired: 15 in]
            n108 = call "sc5511a_get_device_status.vi"("deviceHandle"=w281, "error in"=w280) -> ("deviceHandle"=w282:u32, "Device Status"=w279:T11, "error out"=w283:errorcluster)  [unwired: 15 in]
          }
          event "ALC MODE": Value Change {
            n109 = event-data() -> ("NewVal"=w294:u8)  [unwired: 1 in, 4 out]
            n110 = call "sc5511a_set_alc_mode.vi"("deviceHandle"=w295, "alc mode"=w294, "error in"=w296) -> ("deviceHandle"=w290:u32, "error out"=w292:errorcluster)  [unwired: 15 in]
            n111 = call "sc5511a_get_device_status.vi"("deviceHandle"=w290, "error in"=w292) -> ("deviceHandle"=w291:u32, "Device Status"=w289:T11, "error out"=w293:errorcluster)  [unwired: 15 in]
          }
          event "RF Enable": Value Change {
            n112 = event-data() -> ("NewVal"=w303:bool)  [unwired: 1 in, 4 out]
            n113 = Boolean To (0,1)(Boolean=w303) -> (0, 1=w304:i16)
            n114 = call "sc5511a_set_output.vi"("deviceHandle"=w305, "RF Output"=w304, "error in"=w306) -> ("deviceHandle"=w299:u32, "error out"=w301:errorcluster)  [unwired: 15 in]
            n115 = call "sc5511a_get_device_status.vi"("deviceHandle"=w299, "error in"=w301) -> ("deviceHandle"=w300:u32, "Device Status"=w298:T11, "error out"=w302:errorcluster)  [unwired: 15 in]
          }
          event "SelfCal": Value Change {
            n116 = event-data() -> ("NewVal"=w313:bool)  [unwired: 1 in, 4 out]
            n117 = case shown="True" w313 {
              tunnel: w312 -> [w315 w323]
              tunnel: w311 -> [w314 w322]
              tunnel: [w315 w321] -> w308
              tunnel: [w314 w318] -> w309
              frame False {
              }
              frame True {
                n118 = call "sc5511a_synth_self_cal.vi"("deviceHandle"=w323, "error in"=w322) -> ("deviceHandle"=w321:u32, "error out"=w320:errorcluster)  [unwired: 16 in]
                n119 = call "Time Delay4"("error in (no error)"=w320, "Delay Time (s)"=5.0) -> ("error out"=w319:errorcluster)  [unwired: 9 in]
                n120 = property on="SelfCal" class="Bool (strict)"(error in=w319, "Value"=FALSE ("SelfCal")) -> (error out=w318:errorcluster)  [unwired: 1 in, 1 out]
              }
            }
          }
          event "Power": Value Change {
            n121 = event-data() -> ("NewVal"=w324:sgl)  [unwired: 1 in, 4 out]
            n122 = call "sc5511a_set_level.vi"("deviceHandle"=w327, "level (dBm)"=w324, "error in"=w328) -> ("deviceHandle"=w326:u32, "error out"=w325:errorcluster)  [unwired: 15 in]
          }
          event "GetStatus": Value Change {
            n123 = event-data() -> ("NewVal"=w336:bool)  [unwired: 1 in, 4 out]
            n124 = case shown="True" w336 {
              selector: w336 -> [w342 w345]
              tunnel: w337 -> [w344 w348]
              tunnel: [w339 w347] -> w335
              tunnel: [w342 w345] -> _
              frame True {
                n125 = property on="RF Frequency" class="DigNum (strict)"(error in=w344, "DisabledEnum"=T8."Enabled" ("Disabled")) -> (error out=w340:errorcluster)  [unwired: 1 in, 1 out]
                n126 = property on="Interval (s)" class="DigNum (strict)"(error in=w340, "DisabledEnum"=T8."Enabled" ("Disabled")) -> (error out=w339:errorcluster)  [unwired: 1 in, 1 out]
              }
              frame False {
                n127 = property on="Interval (s)" class="DigNum (strict)"(error in=w348, "DisabledEnum"=T8."Disabled and Grayed Out" ("Disabled")) -> (error out=w347:errorcluster)  [unwired: 1 in, 1 out]
              }
            }
            n128 = call "sc5511a_get_device_status.vi"("deviceHandle"=w332, "error in"=w335) -> ("deviceHandle"=w333:u32, "Device Status"=w331:T11, "error out"=w334:errorcluster)  [unwired: 15 in]
          }
          event "stop": Value Change {
            n129 = event-data() -> ()  [unwired: 1 in, 5 out]
            n130 = property on="stop" class="Bool (strict)"(error in=w350, "Value"=FALSE ("stop")) -> (error out=w351:errorcluster)  [unwired: 1 in, 1 out]
          }
          event "Trigger": Value Change {
            (unwired) u16 0 ("ListMode State")
            n131 = event-data() -> ()  [unwired: 1 in, 5 out]
            n132 = Unbundle By Name(w360) -> ("Operate Status.RF Mode"=w368:u8, "Operate Status.ListRuning"=w367:u8, "List Mode Config.Trigger Source"=w366:u8)
            n133 = case shown="1" w368 {
              tunnel: w367 -> [_ w380]
              tunnel: w366 -> [_ w379]
              tunnel: w365 -> [w371 w378]
              tunnel: [w370 w377] -> w362
              tunnel: w364 -> [w374 w376]
              tunnel: [w374 w375] -> w356
              frame 0, Default {
                n134 = property on="message" class="Str"(error in=w371, "Visible"=TRUE, "Value"="List/Sweep Mode Disabled" ("hwtrigSel'd")) -> (error out=w370:errorcluster)  [unwired: 1 in, 1 out]
              }
              frame 1 {
                n135 = case shown="0, Default" w380 {
                  tunnel: w379 -> [w385 _]
                  tunnel: w378 -> [w384 w397]
                  tunnel: [w383 w396] -> w377
                  tunnel: w376 -> [w382 w398]
                  tunnel: [w381 w395] -> w375
                  frame 0, Default {
                    n136 = case shown="1" w385 {
                      tunnel: [w388 w393] -> w383
                      tunnel: w384 -> [w389 w394]
                      tunnel: w382 -> [w387 w390]
                      tunnel: [w386 w390] -> w381
                      frame 0, Default {
                        n137 = call "sc5511a_list_soft_trigger.vi"("deviceHandle"=w387, "error in"=w389) -> ("deviceHandle"=w386:u32, "error out"=w388:errorcluster)  [unwired: 16 in]
                      }
                      frame 1 {
                        n138 = property on="message" class="Str"(error in=w394, "Visible"=TRUE, "Value"="Requires Hardware Tigger " ("hwtrigSel'd")) -> (error out=w393:errorcluster)  [unwired: 1 in, 1 out]
                      }
                    }
                  }
                  frame 1 {
                    n139 = call "sc5511a_list_soft_trigger.vi"("deviceHandle"=w398, "error in"=w397) -> ("deviceHandle"=w395:u32, "error out"=w396:errorcluster)  [unwired: 16 in]
                  }
                }
              }
            }
            n140 = call "Time Delay"("error in (no error)"=w362) -> ("error out"=w361:errorcluster)  [unwired: 10 in]
            n141 = property on="Trigger" class="Bool (strict)"(error in=w361, "Value"=FALSE ("Soft Tigger")) -> (error out=w358:errorcluster)  [unwired: 1 in, 1 out]
            n142 = call "sc5511a_get_device_status.vi"("deviceHandle"=w356, "error in"=w358) -> ("deviceHandle"=w357:u32, "Device Status"=w355:T11, "error out"=w359:errorcluster)  [unwired: 15 in]
          }
          event "Load Config", "Set As Default": Value Change {
            (unwired) u16 0 ("Direction")
            w409 = FALSE ("Soft Tigger")
            n143 = event-data() -> ()  [unwired: 1 in, 5 out]
            n144 = property on="List Mode Config" class="Clust (strict)"(error in=w435) -> (error out=w434:errorcluster, "Value"=w433:T4)  [unwired: 1 in, 1 out]
            n145 = call "sc5511a_list_mode_config.vi"("deviceHandle"=w436, "List Mode Config"=w433, "error in"=w434) -> ("deviceHandle"=w429:u32, "error out"=w432:errorcluster)  [unwired: 15 in]
            n146 = property on="Sweep Freq Parameter" class="Clust (strict)"(error in=w432) -> (error out=w426:errorcluster, "Value"=w431:T3)  [unwired: 1 in, 1 out]
            n147 = Unbundle(w431) -> ("Start Frequency"=w430:u64, "Stop Frequency"=w423:u64, "Step Frequency"=w422:u64)
            n148 = call "sc5511a_list_start_freq.vi"("deviceHandle"=w429, "List Start frequency"=w430, "error in"=w426) -> ("deviceHandle"=w428:u32, "error out"=w425:errorcluster)  [unwired: 15 in]
            n149 = call "sc5511a_list_stop_freq.vi"("deviceHandle"=w428, "RF frequency"=w423, "error in"=w425) -> ("deviceHandle"=w427:u32, "error out"=w424:errorcluster)  [unwired: 15 in]
            n150 = call "sc5511a_list_step_freq.vi"("deviceHandle"=w427, "List Step Frequency"=w422, "error in"=w424) -> ("deviceHandle"=w416:u32, "error out"=w421:errorcluster)  [unwired: 15 in]
            n151 = property on="Sweep/List Cycles" class="DigNum (strict)"(error in=w421) -> (error out=w419:errorcluster, "Value"=w420:u32)  [unwired: 1 in, 1 out]
            n152 = call "sc5511a_list_cycle_count.vi"("deviceHandle"=w416, "List Cycles"=w420, "error in"=w419) -> ("deviceHandle"=w415:u32, "error out"=w418:errorcluster)  [unwired: 15 in]
            n153 = property on="Dwell Period (ms)" class="DigNum (strict)"(error in=w418) -> (error out=w417:errorcluster, "Value"=w414:dbl)  [unwired: 1 in, 1 out]
            n154 = Multiply(x=w414, y=2.0) -> (x*y=w403:dbl)
            n155 = To Unsigned Long Integer(number=w403) -> (unsigned 32bit integer=w402:u32)
            n156 = call "sc5511a_list_dwell_time.vi"("deviceHandle"=w415, "List Dwell Time"=w402, "error in"=w417) -> ("deviceHandle"=w399:u32, "error out"=w400:errorcluster)  [unwired: 15 in]
            n157 = property on="Set As Default" class="Bool (strict)"(error in=w400) -> (error out=w413:errorcluster, "Value"=w411:bool)  [unwired: 1 in, 1 out]
            n158 = case shown="True" w411 {
              tunnel: w413 -> [w438 w442]
              tunnel: [w438 w441] -> w405
              tunnel: w399 -> [w437 w440]
              tunnel: [w437 w439] -> w412
              frame False {
              }
              frame True {
                n159 = call "sc5511a_store_default_state.vi"("deviceHandle"=w440, "error in"=w442) -> ("deviceHandle"=w439:u32, "error out"=w441:errorcluster)  [unwired: 16 in]
              }
            }
            n160 = call "Time Delay3"("error in (no error)"=w405) -> ("error out"=w404:errorcluster)  [unwired: 10 in]
            n161 = property on="Load Config" class="Bool (strict)"(error in=w404, "Value"=w409) -> (error out=w406:errorcluster)  [unwired: 1 in, 1 out]
            n162 = property on="Set As Default" class="Bool (strict)"(error in=w406, "Value"=w409) -> (error out=w410:errorcluster)  [unwired: 1 in, 1 out]
          }
          event "Download to Buffer": Value Change {
            n163 = event-data() -> ()  [unwired: 1 in, 5 out]
            n164 = Unbundle By Name(w444) -> ("Operate Status.RF Mode"=w443:u8)
            n165 = case shown="0, Default" w443 {
              selector: w443 -> [w453 w489]
              tunnel: w452 -> [w464 w487]
              tunnel: w451 -> [w463 w488]
              tunnel: [w461 w488] -> w450
              tunnel: [w460 w486] -> w446
              tunnel: [w453 w489] -> _
              frame 0, Default {
                # "0xFFFFFFFFFF to end buffer write"
                # "0 to reset the buffer to starting address\nand enable buffer write"
                n166 = call "sc5511a_list_buffer_write.vi"("deviceHandle"=w463, "List Frequency"=u64 0 ("Frequency"), "error in"=w464) -> ("deviceHandle"=w456:u32, "error out"=w459:errorcluster)  [unwired: 15 in]
                n167 = property on="Frequency List (2048 max)" class="Arr (strict)"(error in=w459) -> (error out=w457:errorcluster, "Value"=w458:u64[])  [unwired: 1 in, 1 out]
                n168 = for {
                  tunnel: w458 -> [w470] mode=indexing
                  tunnel: w457 -> [w472]
                  tunnel: w456 -> [w471]
                  tunnel: [w469] -> w454
                  tunnel: [w468] -> w455
                  i -> [w466]
                  stop <- w467 stop-if-true
                  n169 = Greater?(x=w466, y=2048) -> (0:w467:bool)
                  n170 = case shown="False" w467 {
                    tunnel: w472 -> [w481 w483]
                    tunnel: [w476 w483] -> w468
                    tunnel: w471 -> [w480 w482]
                    tunnel: w470 -> [w479 _]
                    tunnel: [w478 w482] -> w469
                    tunnel: w466 -> [w475 _]
                    frame False {
                      n171 = call "sc5511a_list_buffer_write.vi"("deviceHandle"=w480, "List Frequency"=w479, "error in"=w481) -> ("deviceHandle"=w478:u32, "error out"=w477:errorcluster)  [unwired: 15 in]
                      n172 = Increment(x=w475) -> (x+1=w474:i32)
                      n173 = property on="List Points" class="DigNum (strict)"(error in=w477, "Value"=w474) -> (error out=w476:errorcluster)  [unwired: 1 in, 1 out]
                    }
                    frame True {
                    }
                  }
                }
                n174 = call "sc5511a_list_buffer_write.vi"("deviceHandle"=w454, "List Frequency"=u64 1099511627775 ("Frequency"), "error in"=w455) -> ("deviceHandle"=w461:u32, "error out"=w460:errorcluster)  [unwired: 15 in]
              }
              frame 1 {
                n175 = property on="message 2" class="Str"(error in=w487, "Value"="List/Sweep On" ("message 2"), "Visible"=TRUE) -> (error out=w486:errorcluster)  [unwired: 1 in, 1 out]
              }
            }
            n176 = call "Time Delay2"("error in (no error)"=w446) -> ("error out"=w445:errorcluster)  [unwired: 10 in]
            n177 = property on="Download to Buffer" class="Bool (strict)"(error in=w445, "Value"=FALSE ("Download to Buffer")) -> (error out=w449:errorcluster)  [unwired: 1 in, 1 out]
          }
          event "Save Buffer to EEPROM", "Read EEPROM to Buffer": Value Change {
            w495 = FALSE ("Copy EEPROM to Buffer")
            n178 = event-data() -> ()  [unwired: 1 in, 5 out]
            n179 = Unbundle By Name(w491) -> ("Operate Status.RF Mode"=w490:u8)
            n180 = case shown="0, Default" w490 {
              tunnel: w499 -> [w505 w549]
              tunnel: w498 -> [w504 w551]
              tunnel: [w501 w550] -> w497
              tunnel: [w500 w551] -> w493
              frame 0, Default {
                n181 = property on="Read EEPROM to Buffer" class="Bool (strict)"(error in=w505) -> (error out=w502:errorcluster, "Value"=w503:bool)  [unwired: 1 in, 1 out]
                n182 = case shown="True" w503 {
                  tunnel: w504 -> [w519 w545]
                  tunnel: w502 -> [w513 w544]
                  tunnel: [w515 w543] -> w501
                  tunnel: [w517 w542] -> w500
                  frame True {
                    w520 = u16 1 items=["Buffer to EEPROM", "EEPROM to Buffer"] ("List Eeprom Config")
                    n183 = property on="List Points" class="DigNum (strict)"(error in=w513) -> (error out=w512:errorcluster, "Value"=w511:u32)  [unwired: 1 in, 1 out]
                    n184 = call "sc5511a_list_buffer_transfer.vi"("deviceHandle"=w519, "transfer mode"=w520, "error in"=w512) -> ("deviceHandle"=w516:u32, "error out"=w518:errorcluster)  [unwired: 15 in]
                    n185 = Greater Than 0?(x=w511) -> (x > 0?=w510:bool)
                    n186 = case shown="True" w510 {
                      tunnel: w518 -> [w523 w533]
                      tunnel: [w525 w532] -> w517
                      tunnel: w516 -> [w525 w531]
                      tunnel: [w523 w530] -> w514
                      tunnel: [u64[] [] w529] -> w509
                      tunnel: w511 -> [_ w528]
                      tunnel: [0 w527] -> w506
                      tunnel: [0 ("length") 1 ("length")] -> w508
                      frame False {
                      }
                      frame True {
                        n187 = while {
                          tunnel: w533 -> [w541]
                          tunnel: [w540] -> w530
                          tunnel: [w539] -> w532
                          tunnel: w531 -> [w538]
                          tunnel: [w537] -> w529 mode=indexing
                          tunnel: w528 -> [w536]
                          tunnel: [w534] -> w527
                          i -> [w534]
                          stop <- w535 continue-if-true
                          n188 = Less?(x=w534, y=w536) -> (x < y?=w535:bool)
                          n189 = call "sc5511a_list_buffer_read.vi"("deviceHandle"=w538, "address"=w534, "error in"=w541) -> ("deviceHandle"=w539:u32, "frequency"=w537:u64, "error out"=w540:errorcluster)  [unwired: 14 in]
                        }
                      }
                    }
                    n190 = Delete From Array(array=w509, length=w508, index=w506) -> (array with subset deleted=w507:u64[])  [unwired: 1 out]
                    n191 = property on="List Points" class="DigNum (strict)"("Value"=w506) -> ()  [unwired: 2 in, 2 out]
                    n192 = property on="Frequency List (2048 max)" class="Arr (strict)"(error in=w514, "Value"=w507) -> (error out=w515:errorcluster)  [unwired: 1 in, 1 out]
                  }
                  frame False {
                    w546 = u16 0 items=["Buffer to EEPROM", "EEPROM to Buffer"] ("List Eeprom Config")
                    n193 = call "sc5511a_list_buffer_transfer.vi"("deviceHandle"=w545, "transfer mode"=w546, "error in"=w544) -> ("deviceHandle"=w542:u32, "error out"=w543:errorcluster)  [unwired: 15 in]
                  }
                }
              }
              frame 1 {
                n194 = property on="message 2" class="Str"(error in=w549, "Value"="List Mode On" ("message 2"), "Visible"=TRUE) -> (error out=w550:errorcluster)  [unwired: 1 in, 1 out]
              }
            }
            n195 = property on="Read EEPROM to Buffer" class="Bool (strict)"(error in=w497, "Value"=w495) -> (error out=w496:errorcluster)  [unwired: 1 in, 1 out]
            n196 = property on="Save Buffer to EEPROM" class="Bool (strict)"(error in=w496, "Value"=w495) -> (error out=w494:errorcluster)  [unwired: 1 in, 1 out]
          }
        }
        n197 = Greater?(x=w157, y=u32 1500) -> (0:w155:bool)
        n198 = Multiply(x=w153, y=u16 1000) -> (x*y=w151:u16)
        n199 = Greater?(x=w152, y=w151) -> (0:w105:bool)
        n200 = local read "GetStatus"() -> (w149:bool)
        n201 = And(x=w149, y=w105) -> (x .and. y?=w103:bool)
        n202 = Unbundle By Name(w108) -> ("Operate Status.ListRuning"=w107:u8)
        n203 = case shown="True" w103 {
          tunnel: w160 -> [w183 w188]
          tunnel: w159 -> [w182 w187]
          tunnel: [w182 w185] -> w110
          tunnel: [w183 w186] -> w112
          tunnel: [w181 w184] -> w119
          tunnel: w108 -> [w181 _]
          frame False {
          }
          frame True {
            n204 = call "sc5511a_get_device_status.vi"("deviceHandle"=w188, "error in"=w187) -> ("deviceHandle"=w186:u32, "Device Status"=w184:T11, "error out"=w185:errorcluster)  [unwired: 15 in]
          }
        }
        n205 = Not Equal To 0?(x=w107) -> (x != 0?=w106:bool)
        n206 = And(x=w106, y=w105) -> (x .and. y?=w104:bool)
        n207 = Unbundle By Name(w119) -> ("Operate Status.Lock Mode"=w133:u8, "Operate Status.RFOutState"=w123:u8, "Operate Status.AutoPwrLevel"=w124:u8, "Operate Status.AlcMode"=w125:u8, "Operate Status.RF1 Standby"=w126:u8, "Operate Status.RF Mode"=w127:u8, "Operate Status.ListRuning"=w116:u8, "Operate Status.RF2 Standby"=w128:u8, "Operate Status.Ref Lock Enable"=w129:u8, "Operate Status.ExtRefDetected"=w130:u8, "Operate Status.RefOutSelect"=w131:u8, "PLL Status.Sum PLL"=w132:u8, "PLL Status.Crs assist PLL"=w137:u8, "PLL Status.Crs PLL"=w138:u8, "PLL Status.Crs Ref PLL"=w136:u8, "PLL Status.Fine PLL"=w140:u8, "Operate Status.Device Accessed"=w141:u8, "Operate Status.OverTempStatus"=w142:u8)
        n208 = case shown="True" w104 {
          tunnel: [w165 w172] -> w114
          tunnel: w115 -> [w165 _]
          tunnel: w113 -> [_ w172]
          tunnel: w112 -> [w164 w171]
          tunnel: [w164 w170] -> w111
          tunnel: w110 -> [w163 w169]
          tunnel: [w163 w167] -> w109
          frame False {
          }
          frame True {
            n209 = call "sc5511a_get_temperature.vi"("deviceHandle"=w171, "error in"=w169) -> ("deviceHandle"=w170:u32, "temperature"=w166:sgl, "error out"=w168:errorcluster)  [unwired: 15 in]
            n210 = property on="Temperature" class="DigNum (strict)"(error in=w168, "Value"=w166) -> (error out=w167:errorcluster)  [unwired: 1 in, 1 out]
          }
        }
        n211 = case shown="True" w155 {
          selector: w155 -> [_ w177]
          tunnel: w109 -> [w174 w180]
          tunnel: [w174 w179] -> w144
          tunnel: w147 -> [w173 _]
          tunnel: [w173 w175] -> w148
          tunnel: w113 -> [_ w175]
          frame False {
          }
          frame True {
            n212 = Not(x=w177) -> (.not. x?=w176:bool)
            n213 = property on="message" class="Str"(error in=w180, "Visible"=w176) -> (error out=w178:errorcluster)  [unwired: 1 in, 1 out]
            n214 = property on="message 2" class="Str"(error in=w178, "Visible"=w176) -> (error out=w179:errorcluster)  [unwired: 1 in, 1 out]
          }
        }
        n215 = Not Equal To 0?(x=w133) -> (x != 0?=w134:bool)
        n216 = Select(t=w137, s=w134, f=w138) -> (s? t:f=w135:u8)
        n217 = And(x=w135, y=w136) -> (x .and. y?=w139:u8)
        n218 = Not Equal To 0?(x=w132) -> (x != 0?=w120:bool)
        n219 = Not Equal To 0?(x=w139) -> (x != 0?=w121:bool)
        n220 = Not Equal To 0?(x=w140) -> (x != 0?=w122:bool)
        n221 = Unbundle By Name(w144) -> ("status"=w145:bool)
        n222 = Bundle By Name(cluster=T9 {"Synth Mode"=0, "RF Out"=0, "Auto Power"=0, "ALC Mode"=0, "Standby"=0, "Rf RF Mode"=0, "List Mode State"=0, "RF2 Standby"=0, "Ref Lock Enable"=0, "Ext Ref Detected"=0, "Ref out mode"=0, "Main PLL"=1, "Crs PLL"=1, "Fine PLL"=1, "device accessed"=0, "Over Temp"=0, "MainLED"=FALSE, "CrsLED"=FALSE, "FineLED"=FALSE} ("Device Status"), "Synth Mode"=w133, "RF Out"=w123, "Auto Power"=w124, "ALC Mode"=w125, "Standby"=w126, "Rf RF Mode"=w127, "List Mode State"=w116, "RF2 Standby"=w128, "Ref Lock Enable"=w129, "Ext Ref Detected"=w130, "Ref out mode"=w131, "Main PLL"=w132, "Crs PLL"=w139, "Fine PLL"=w140, "device accessed"=w141, "Over Temp"=w142, "MainLED"=w120, "CrsLED"=w121, "FineLED"=w122) -> (w118:T9)
        n223 = Or(x=w145, y=w146) -> (x .or. y?=w143:bool)
        n224 = property on="Device Status" class="Clust (strict)"("Value"=w118) -> ()  [unwired: 2 in, 2 out]
      }
      n225 = call "sc5511a_close_device.vi"("deviceHandle"=w93, "error in (no error)"=w94) -> ("error out"=w92:errorcluster)  [unwired: 17 in]
    }
    frame Error {
    }
  }
  n226 = Unbundle By Name(w7) -> ("status"=w3:bool)
  n227 = case shown="True" w3 {
    selector: w3 -> [_ w553]
    frame False {
    }
    frame True {
      n228 = property on="error out" class="Clust (strict)"("Visible"=w553) -> ()  [unwired: 2 in, 2 out]
      n229 = property on="Tab Control" class="TabCtl (strict)"("Value"=T1."Device Info" ("Tab Control")) -> ()  [unwired: 2 in, 2 out]
    }
  }
  n230 = property on="On" class="Bool (strict)"(error in=w7, "Value"=FALSE ("Visible")) -> (error out=→"error out":errorcluster)  [unwired: 1 in, 1 out]
